vi "thcd401_read_current.vi"(8 "error in":errorcluster, 11 "conn_id_in":refnum<k5>) -> (0 "error out":errorcluster, 1 "mode_array":i32[](array[numeric]), 2 "value_array":dbl[](array[numeric]), 3 "conn_id_out":refnum<k5>, 4 "status":bool)   [LabVIEW 2019]
panel:
  out "modes":i32
  out "string":string
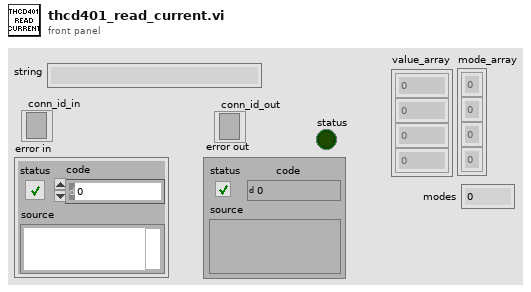
[diagram p1: front panel]
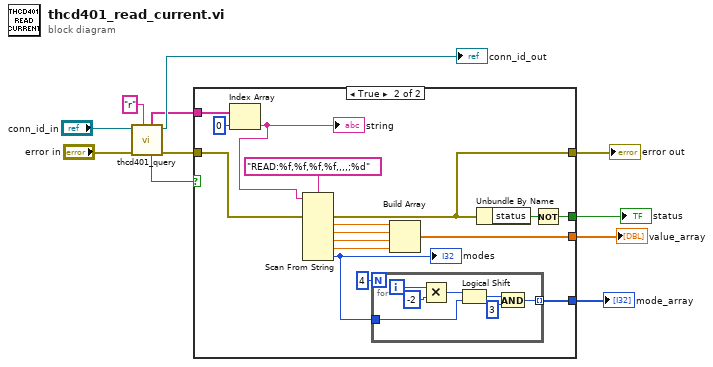
[diagram p0: block diagram]
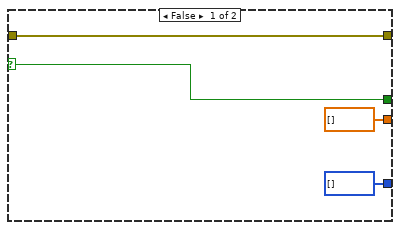
[diagram p2: hidden frame]
diagram:
  n1 = call "thcd401_query.vi"("command"="r" ("string"), "error in"="error in", "conn_id_in"="conn_id_in") -> ("error out"=w6:errorcluster, "conn_id_out"=→"conn_id_out":refnum<k5>, "status"=w3:bool, "data_array"=w7:string[])  [unwired: 5 in]
  n2 = case shown="True" w3 {
    selector: w3 -> [w14 _]
    tunnel: w7 -> [_ w31]
    tunnel: w6 -> [w15 w29]
    tunnel: [dbl[] [] w23] -> w5
    tunnel: [w15 w21] -> w4
    tunnel: [w14 w19] -> w2
    tunnel: [i32[] [] w16] -> w1
    frame False {
    }
    frame True {
      n3 = Index Array(array=w31, index=0 ("length")) -> (element=w22:string)
      "string" <- w22
      n4 = Scan From String(format string="READ:%f,%f,%f,%f,,,,;%d", input string=w22, error in=w29) -> (error out=w21:errorcluster, output 1=w27:dbl, output 2=w26:dbl, output 3=w25:dbl, output 4=w24:dbl, output 5=w17:i32)  [unwired: 6 in, 2 out]
      "modes" <- w17
      n5 = for {
        N: 4 -> [_]
        tunnel: w17 -> [w32]
        tunnel: [w35] -> w16 mode=indexing
        i -> [w34]
        n6 = Multiply(x=w34, y=-2) -> (x*y=w33:i32)
        n7 = Logical Shift(y=w33, x=w32) -> (x << y=w37:i32)
        n8 = And(x=w37, y=3) -> (x .and. y?=w35:i32)
      }
      n9 = Build Array(w27, w26, w25, w24) -> (w23:dbl[])
      n10 = Unbundle By Name(w21) -> ("status"=w20:bool)
      n11 = Not(x=w20) -> (.not. x?=w19:bool)
    }
  }
  "error out" <- w4
  "status" <- w2
  "value_array" <- w5
  "mode_array" <- w1
